vi "Read Message.vi"(8 "error in (no error)":errorcluster, 11 "Example Class in":refnum<class "Example Class.lvclass">) -> (0 "error out":errorcluster, 2 "Message":string, 3 "Example Class out":refnum<class "Example Class.lvclass">)   [LabVIEW 2017, in "Example Class.lvclass"]
uses:
  Example Class.lvclass
  Example Class.lvclass/Example Class.ctl
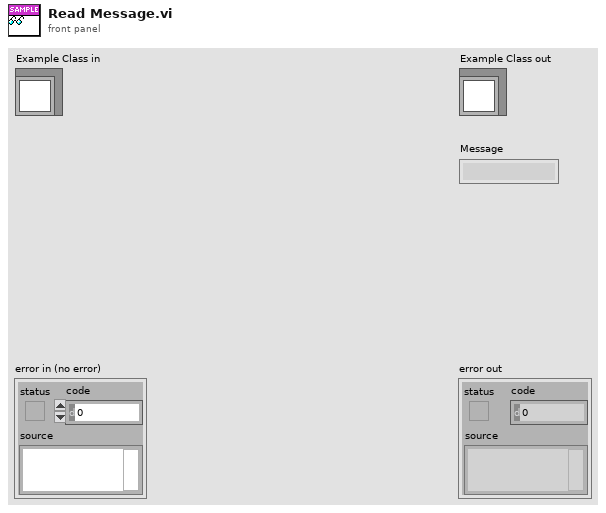
[diagram p1: front panel]
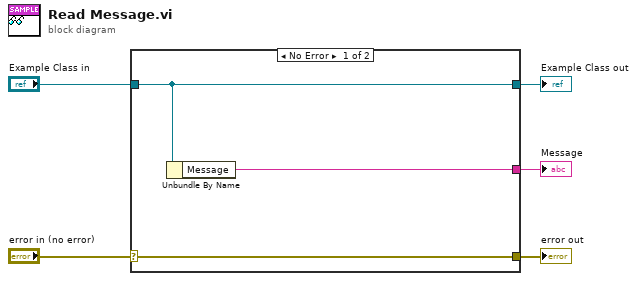
[diagram p0: block diagram]
diagram:
  n1 = case shown="No Error" "error in (no error)" {
    selector: "error in (no error)" -> [w8 w9]
    tunnel: [w8 w9] -> w4
    tunnel: [w7 w10] -> w2
    tunnel: "Example Class in" -> [w7 w10]
    tunnel: [w6 _] -> w1
    frame No Error {
      n2 = Unbundle By Name(w7) -> ("Message"=w6:string)
    }
    frame Error {
    }
  }
  "error out" <- w4
  "Example Class out" <- w2
  "Message" <- w1
